vi "Operation Main.vi"(8 "error in (no error)":errorcluster, 11 "Node Actor in":refnum<class "Node Actor.lvclass">) -> (0 "error out":errorcluster, 3 "Node Actor out":refnum<class "Node Actor.lvclass">)   [LabVIEW 2024, in "Node Actor.lvclass"]
uses:
  Node Actor.lvclass
  Task/Task Ancestor/Task Ancestor.lvclass
  Node Actor.lvclass/Node Actor.ctl
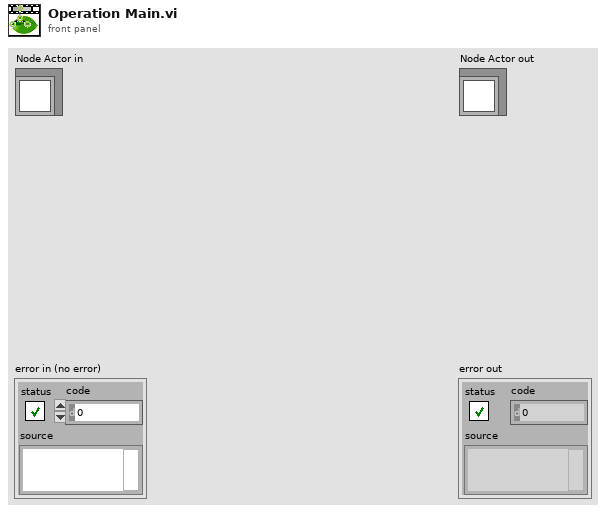
[diagram p1: front panel]
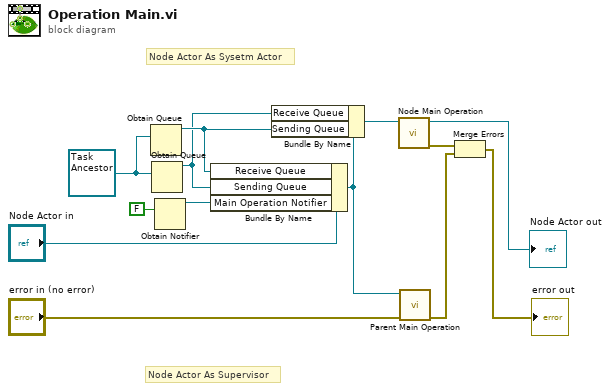
[diagram p0: block diagram]
diagram:
  w11 = refnum<class "Task Ancestor.lvclass"> refnum ("Task Ancestor.lvclass")
  # "Node Actor As Sysetm Actor"
  # "Node Actor As Supervisor"
  n1 = Obtain Queue(element data type=w11) -> (queue out=w7:refnum<queue>)  [unwired: 4 in, 2 out]
  n2 = Obtain Queue(element data type=w11) -> (queue out=w6:refnum<queue>)  [unwired: 4 in, 2 out]
  n3 = Obtain Notifier(notification data type=FALSE) -> (notifier out=w9:refnum<notifier>)  [unwired: 3 in, 2 out]
  n4 = Bundle By Name(cluster="Node Actor in", "Receive Queue"=w7, "Sending Queue"=w6, "Main Operation Notifier"=w9) -> (w8:refnum<class "Node Actor.lvclass">)
  n5 = Bundle By Name(cluster=w8, "Receive Queue"=w6, "Sending Queue"=w7) -> (w5:refnum<class "Node Actor.lvclass">)
  n6 = call-dynamic "Node Main Operation.vi"("Node Actor in"=w5) -> ("error out"=w4:errorcluster, "Node Actor out"=→"Node Actor out":refnum<class "Node Actor.lvclass">)  [unwired: 9 in]
  n7 = call-dynamic "Parent Main Operation.vi"("error in (no error)"="error in (no error)", "Node Actor in"=w8) -> ("error out"=w3:errorcluster)  [unwired: 8 in, 1 out]
  n8 = Merge Errors(w4, w3) -> (→"error out":errorcluster)
